vi "graph_luz_y_temp.vi"() -> ()   [LabVIEW 2021]
panel:
  out "Curva de luz 2":cluster{"Ramp Pattern":dbl[], u32[]}[](graph)
  in  "Luz 5":path
  in  "Temp 4":path
  in  "Temp3":path
  in  "Temp 2":path
  in  "Luz 4":path
  in  "Luz 3":path
  in  "Luz 2":path
  out "Curva de temperatura":cluster{"Ramp Pattern":dbl[], u32[]}[](graph)
  in  "Temp 1":path
  out "Curva de luz":cluster{"Ramp Pattern":dbl[], u32[]}[](graph)
  in  "Luz 1":path
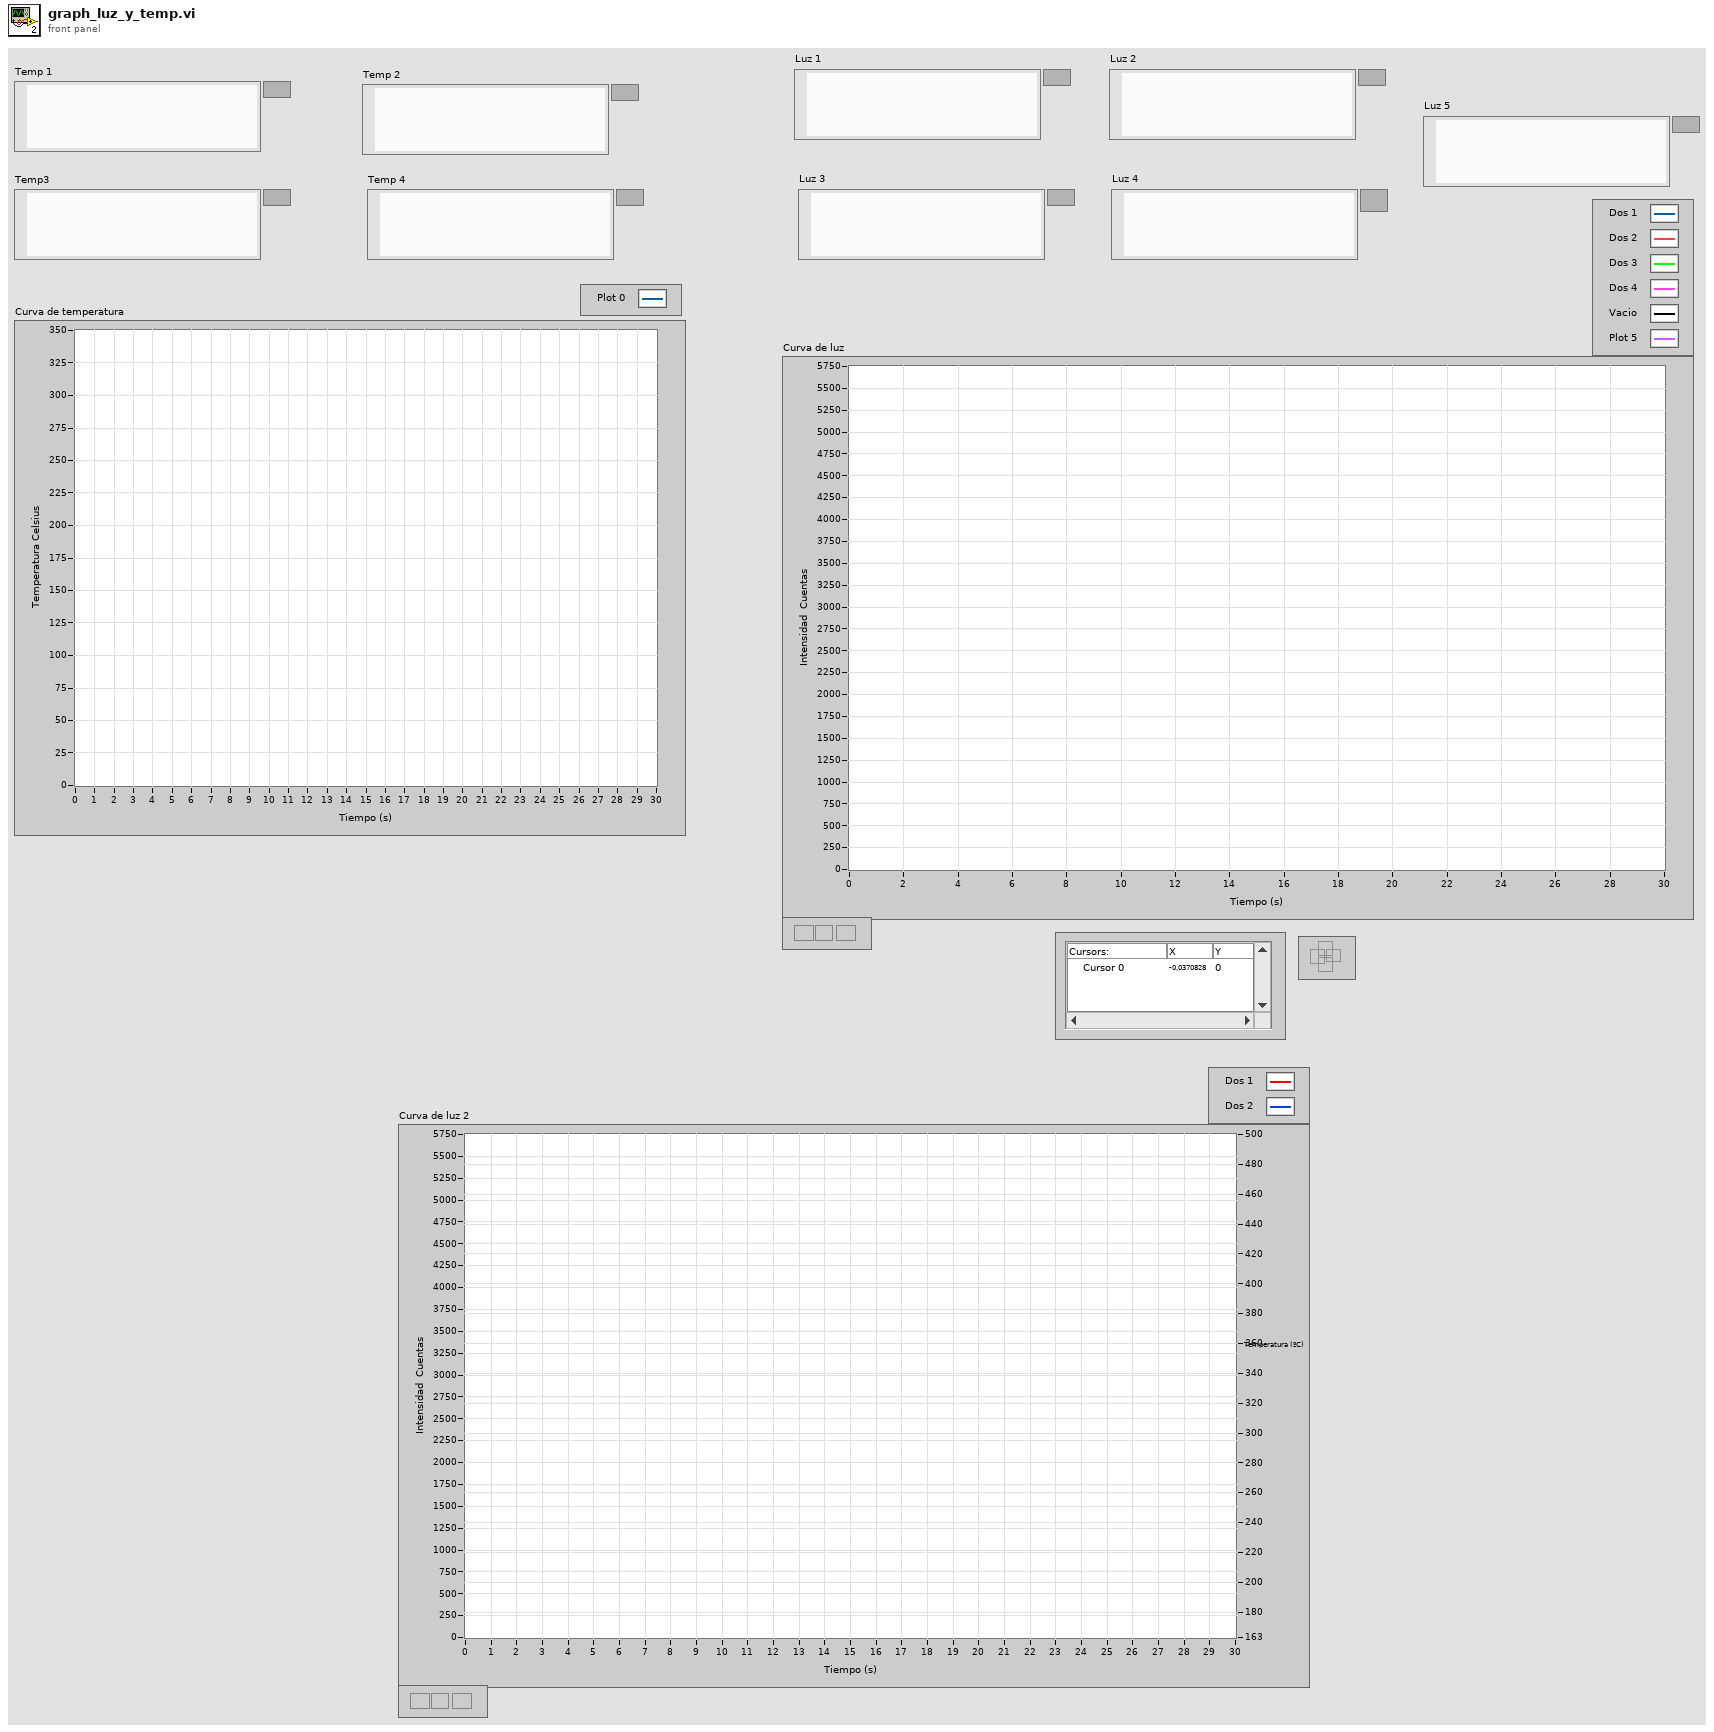
[diagram p1: front panel]
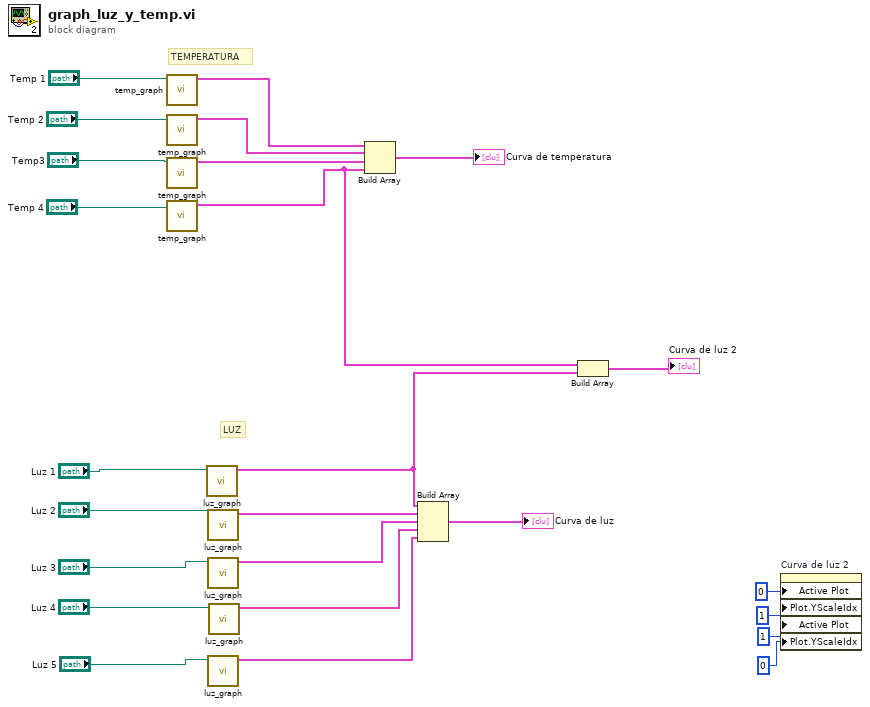
[diagram p0: block diagram]
diagram:
  # "LUZ"
  # "TEMPERATURA"
  n1 = call "temp_graph.vi"("file path (dialog if empty) in"="Temp 1") -> ("Curva de temperatura"=w7:cluster{"Ramp Pattern":dbl[], u32[]})  [unwired: 10 in]
  n2 = call "temp_graph.vi"("file path (dialog if empty) in"="Temp 2") -> ("Curva de temperatura"=w13:cluster{"Ramp Pattern":dbl[], u32[]})  [unwired: 10 in]
  n3 = call "temp_graph.vi"("file path (dialog if empty) in"="Temp3") -> ("Curva de temperatura"=w12:cluster{"Ramp Pattern":dbl[], u32[]})  [unwired: 10 in]
  n4 = call "temp_graph.vi"("file path (dialog if empty) in"="Temp 4") -> ("Curva de temperatura"=w1:cluster{"Ramp Pattern":dbl[], u32[]})  [unwired: 10 in]
  n5 = call "luz_graph.vi"("file path (dialog if empty)"="Luz 1") -> ("Curva de luz"=w3:cluster{"Ramp Pattern":dbl[], u32[]})  [unwired: 10 in]
  n6 = call "luz_graph.vi"("file path (dialog if empty)"="Luz 2") -> ("Curva de luz"=w20:cluster{"Ramp Pattern":dbl[], u32[]})  [unwired: 10 in]
  n7 = call "luz_graph.vi"("file path (dialog if empty)"="Luz 3") -> ("Curva de luz"=w19:cluster{"Ramp Pattern":dbl[], u32[]})  [unwired: 10 in]
  n8 = call "luz_graph.vi"("file path (dialog if empty)"="Luz 5") -> ("Curva de luz"=w10:cluster{"Ramp Pattern":dbl[], u32[]})  [unwired: 10 in]
  n9 = call "luz_graph.vi"("file path (dialog if empty)"="Luz 4") -> ("Curva de luz"=w18:cluster{"Ramp Pattern":dbl[], u32[]})  [unwired: 10 in]
  n10 = Build Array(w7, w13, w12, w1) -> (→"Curva de temperatura":cluster{"Ramp Pattern":dbl[], u32[]}[])
  n11 = Build Array(w3, w20, w19, w18, w10) -> (→"Curva de luz":cluster{"Ramp Pattern":dbl[], u32[]}[])
  n12 = Build Array(w1, w3) -> (→"Curva de luz 2":cluster{"Ramp Pattern":dbl[], u32[]}[])
  n13 = property on="Curva de luz 2" class="XYGraph (strict)"("Active Plot"=u32 0, "Plot.YScaleIdx"=u32 1 ("Plot.Y Scale Index"), "Active Plot"=u32 1, "Plot.YScaleIdx"=u32 0 ("Plot.Y Scale Index")) -> ()  [unwired: 2 in, 2 out]
